vi "Split DMA by Direction.vi"(8 "error in":errorcluster, 11 "DMA configuration array":T1[](array[typedef])) -> (0 "error out":errorcluster, 2 "HostToTarget":T4[](array[typedef]) {"Data Type" format="%.0x"}, 3 "TargetToHost":T4[](array[typedef]) {"Data Type" format="%.0x"})   [LabVIEW 2018, in "FPGA Addon System Explorer.lvlib"]
uses:
  FPGA Addon System Explorer.lvlib
  Addon Shared/Types/DMA Information.ctl
  Addon Shared/Types/Data Type.ctl
  <vilib>/rvi/FIFO/Fifo_Types/Fifo_DMA_Config.ctl
  <vilib>/rvi/DataTransferAndStorage/Container/Common/niFpgaDataTypeControl.ctl
  <vilib>/rvi/ClientSDK/Core/ModuleGeneration/CommunicationInterfaceUtility/niFpgaDmaChannelImplementation.ctl
  Addon Shared/FPGA Addon Shared.lvlib
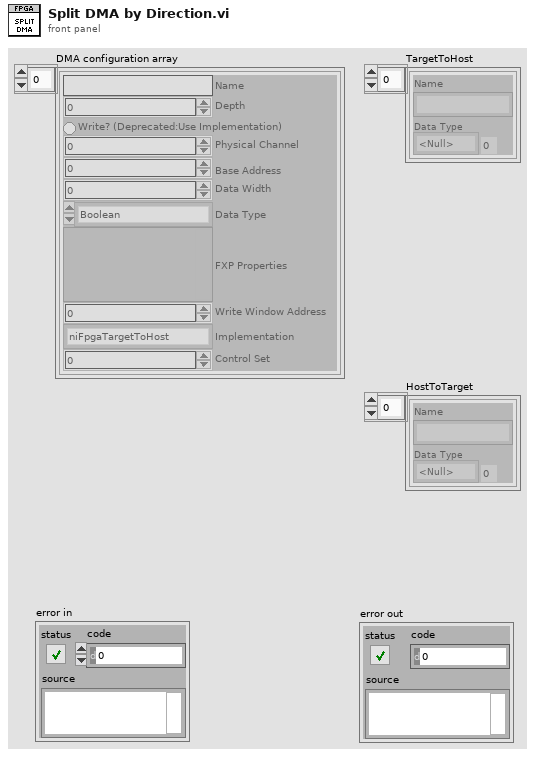
[diagram p1: front panel]
types:
  T1 = typedef "Fifo_DMA_Config.ctl" = cluster{"Name":string, "Depth":u32, "Write? (Deprecated:Use Implementation)":bool, "Physical Channel":u32, "Base Address":u32, "Data Width":u32, "Data Type":T2, "FXP Properties":variant, "Write Window Address":u32, "Implementation":T3, "Control Set":u32}
  T2 = typedef "niFpgaDataTypeControl.ctl" = enum32{"Boolean", "I8", "I16", "I32", "I64", "U8", "U16", "U32", "U64", "FXP", "CustomControl", "SGL"}
  T3 = typedef "niFpgaDmaChannelImplementation.ctl" = enum16{"niFpgaTargetToHost", "niFpgaHostToTarget", "niFpgaPeerToPeerWriter", "niFpgaPeerToPeerReader", "niCoreTargetToHost", "niCoreHostToTarget"}
  T4 = typedef "FPGA Addon Shared.lvlib/DMA Information.ctl" = cluster{"Name":string, "Data Type":T5}
  T5 = typedef "FPGA Addon Shared.lvlib/Data Type.ctl" = enum8{"<Null>", "I8", "I16", "I32", "I64", "U8", "U16", "U32", "U64", "SGL", "Boolean", "Analog PWM In Settings", "Analog PWM In", "Digital PWM In Settings", "Digital PWM In", "Digital PWM Out", "Sine Out", "FXP+/-24.5", "FXP+/-16.5", "FXP+/-32.8", "FXP+/-64.32", "FXP+/-16.7", "FXP+/-20.5", "FXP+/-27.5", "FXP+/-32.16", "FXP+16.3", "FXP+18.3", "Digital Static In", "Digital Static Out", "Digital Static In Settings", "Digital WSS Out", "Quad Encoder Settings", "Quad Encoder In", "Group"}
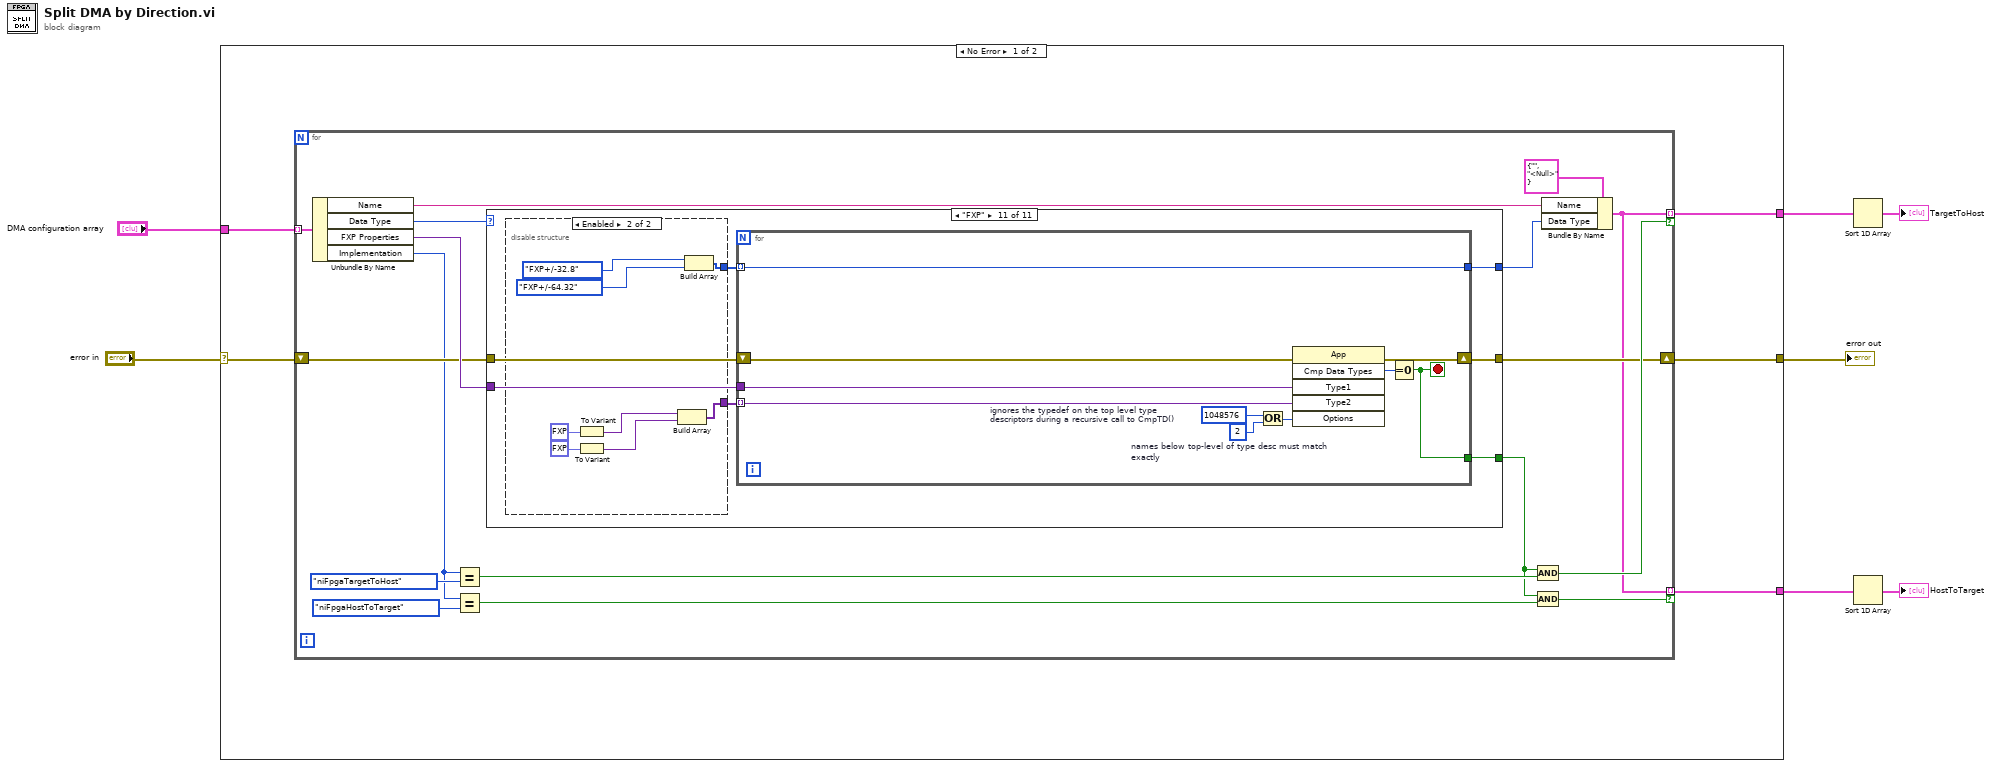
[diagram p0: block diagram]
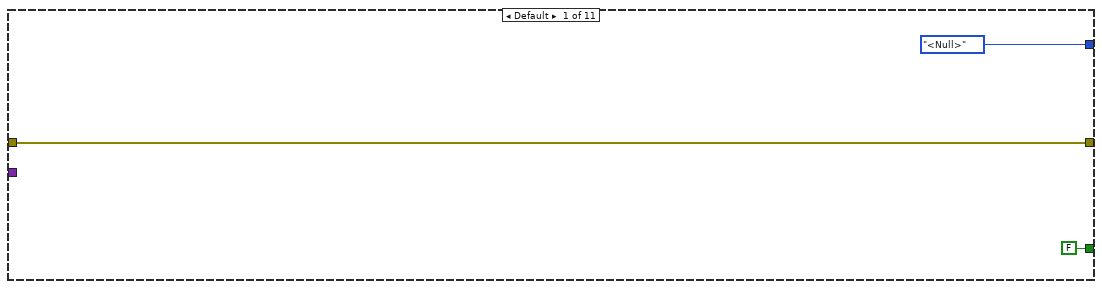
[diagram p2: hidden frame]
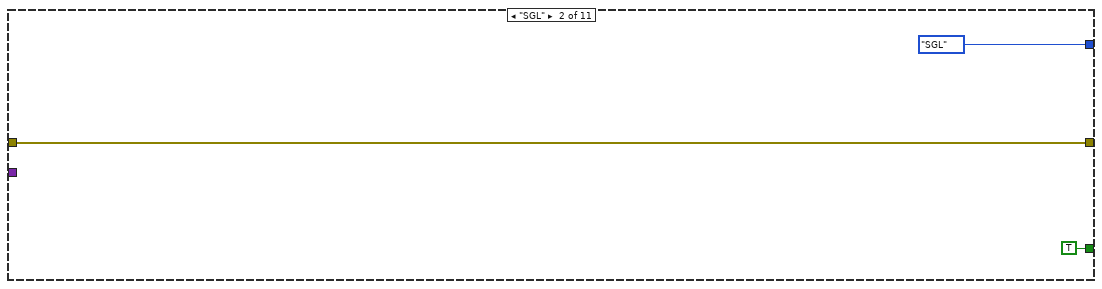
[diagram p3: hidden frame]
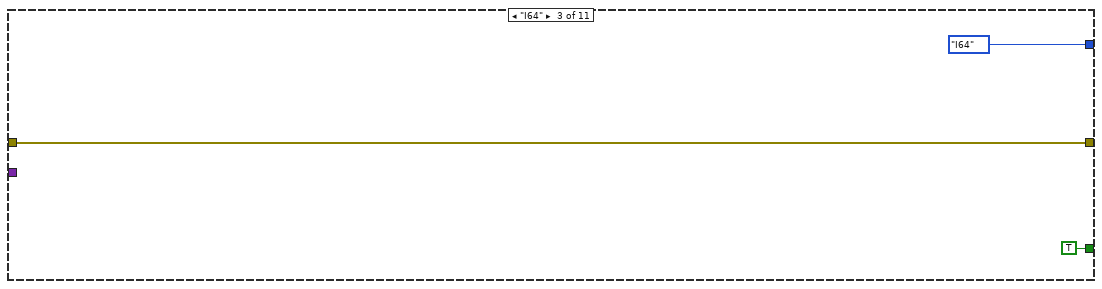
[diagram p4: hidden frame]
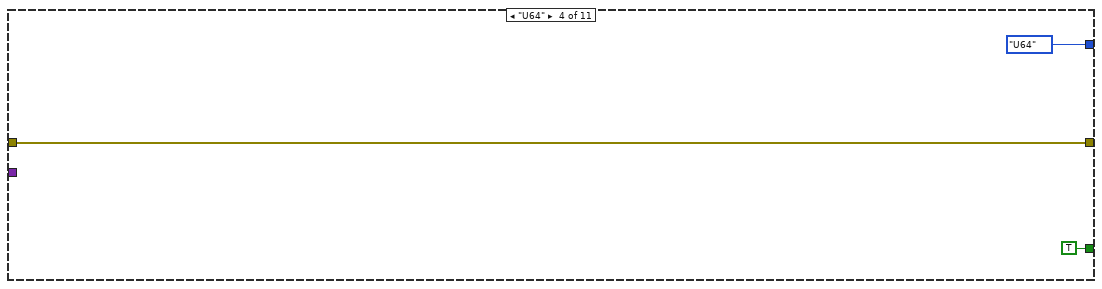
[diagram p5: hidden frame]
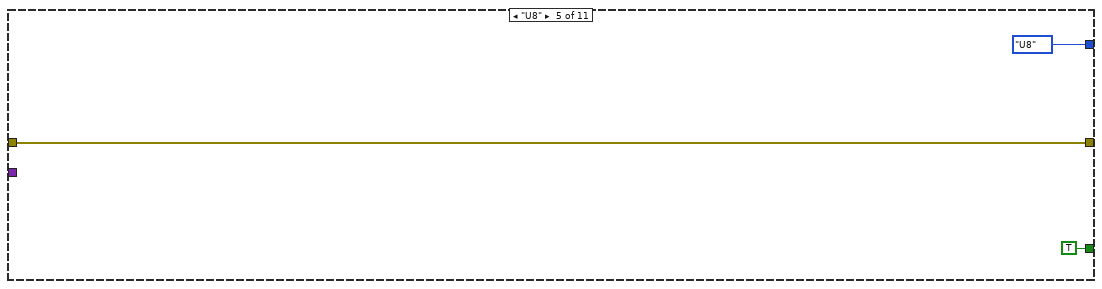
[diagram p6: hidden frame]
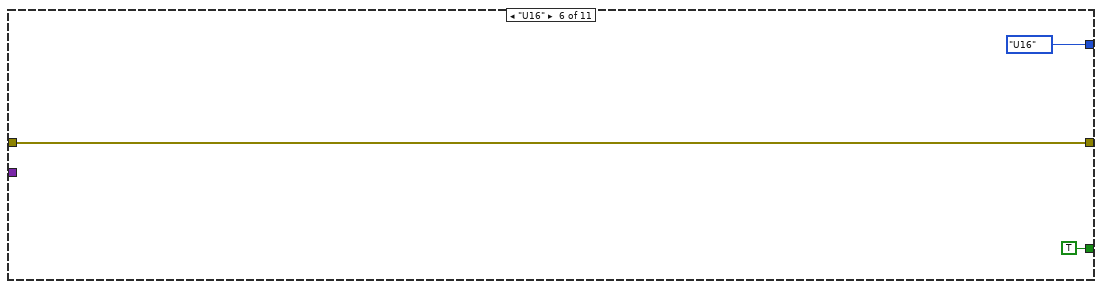
[diagram p7: hidden frame]
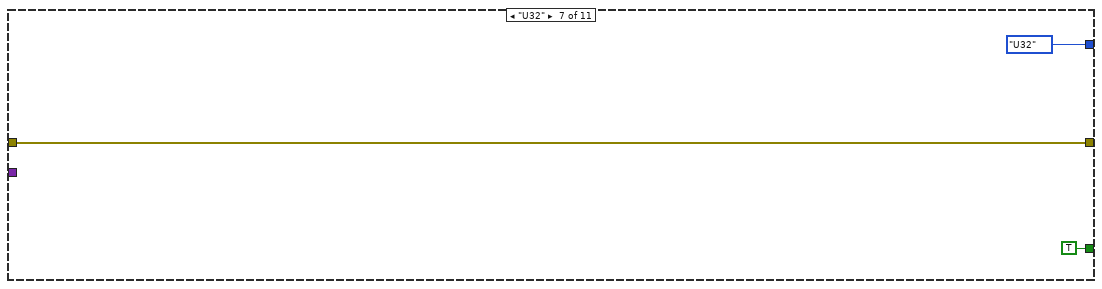
[diagram p8: hidden frame]
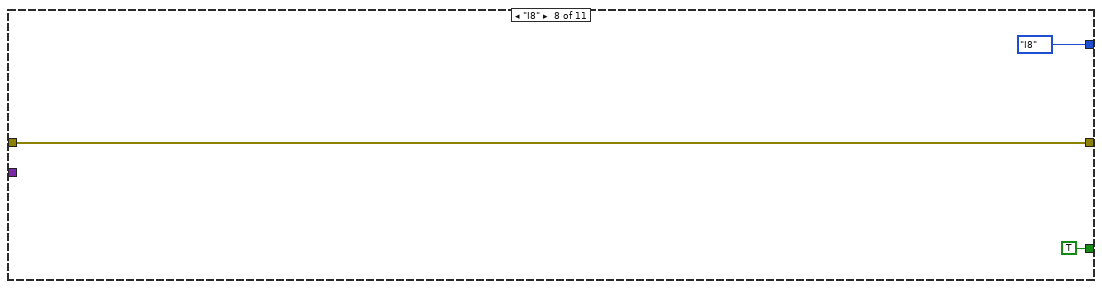
[diagram p9: hidden frame]
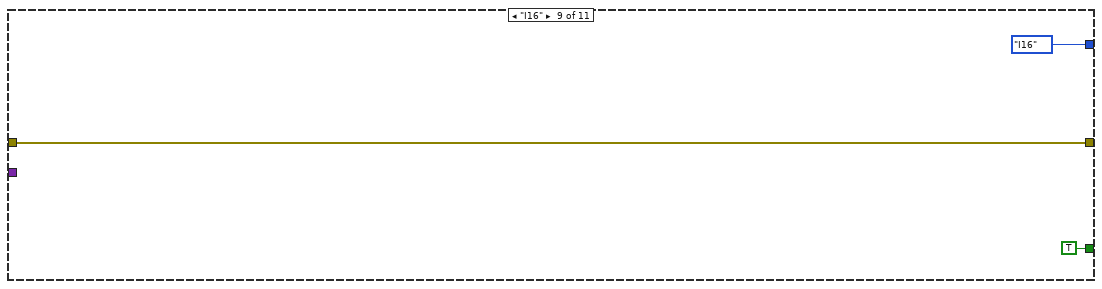
[diagram p10: hidden frame]
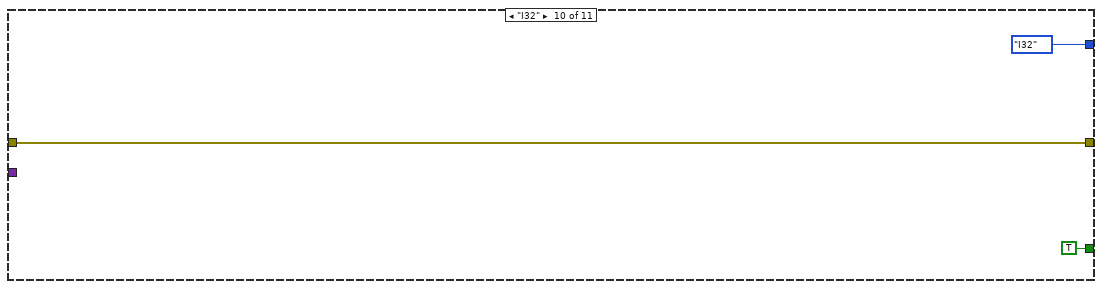
[diagram p11: hidden frame]
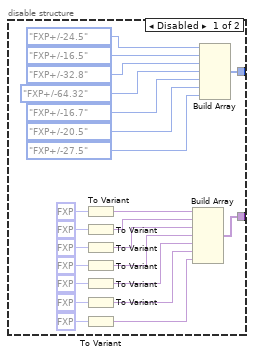
[diagram p12: hidden frame]
diagram:
  n1 = case shown="No Error" "error in" {
    selector: "error in" -> [w8 w108]
    tunnel: "DMA configuration array" -> [w12 _]
    tunnel: [w11 _] -> w5
    tunnel: [w10 _] -> w3
    tunnel: [w9 w108] -> w2
    frame No Error {
      n2 = for {
        tunnel: w12 -> [w15] mode=indexing
        tunnel: [w14] -> w10 mode=indexing if=w26
        tunnel: [w14] -> w11 mode=indexing if=w24
        shift-right: [w22] -> w9
        shift-left: w8 -> [w21]
        n3 = Unbundle By Name(w15) -> ("Name"=w19:string, "Data Type"=w18:T2, "FXP Properties"=w23:variant, "Implementation"=w13:T3)
        n4 = Equal?(x=w13, y=niFpgaDmaChannelImplementation."niFpgaTargetToHost") -> (x = y?=w27:bool)
        n5 = Equal?(x=w13, y=niFpgaDmaChannelImplementation."niFpgaHostToTarget") -> (x = y?=w25:bool)
        n6 = case shown="\"FXP\"" w18 {
          tunnel: w23 -> [_ _ _ _ _ _ _ _ _ _ w66]
          tunnel: [w32 w35 w38 w41 w44 w47 w50 w53 w56 w59 w65] -> w22
          tunnel: w21 -> [w32 w35 w38 w41 w44 w47 w50 w53 w56 w59 w64]
          tunnel: [Data_Type."<Null>" ("Data Type") Data_Type."SGL" ("Data Type") Data_Type."I64" ("Data Type") Data_Type."U64" ("Data Type") Data_Type."U8" ("Data Type") Data_Type."U16" ("Data Type") Data_Type."U32" ("Data Type") Data_Type."I8" ("Data Type") Data_Type."I16" ("Data Type") Data_Type."I32" ("Data Type") w61] -> w17
          tunnel: [FALSE TRUE TRUE TRUE TRUE TRUE TRUE TRUE TRUE TRUE w60] -> w16
          frame Default {
          }
          frame "SGL" {
          }
          frame "I64" {
          }
          frame "U64" {
          }
          frame "U8" {
          }
          frame "U16" {
          }
          frame "U32" {
          }
          frame "I8" {
          }
          frame "I16" {
          }
          frame "I32" {
          }
          frame "FXP" {
            n7 = disable-structure shown="Enabled" {
              disable-tunnel: [w75 w93] -> w63
              disable-tunnel: [w67 w90] -> w62
              frame Disabled {
                n8 = To Variant(anything=fxp<+/-,24,5> 0.0 ("Numeric 1 In")) -> (Variant=w76:variant)
                n9 = To Variant(anything=fxp<+/-,16,5> 0.0 ("Numeric 2 In")) -> (Variant=w77:variant)
                n10 = To Variant(anything=fxp<+/-,32,8> 0.0 ("Numeric 3 In")) -> (Variant=w78:variant)
                n11 = To Variant(anything=fxp<+/-,64,32> 0.0 ("Numeric 4 In")) -> (Variant=w79:variant)
                n12 = To Variant(anything=fxp<+/-,16,7> 0.0 ("Numeric 4 In")) -> (Variant=w85:variant)
                n13 = To Variant(anything=fxp<+/-,20,5> 0.0 ("Numeric 4 In")) -> (Variant=w87:variant)
                n14 = To Variant(anything=fxp<+/-,27,5> 0.0 ("Numeric 4 In")) -> (Variant=w89:variant)
                n15 = Build Array(w76, w77, w78, w79, w85, w87, w89) -> (w75:variant[])
                n16 = Build Array(Data_Type."FXP+/-24.5" ("Data Type"), Data_Type."FXP+/-16.5" ("Data Type"), Data_Type."FXP+/-32.8" ("Data Type"), Data_Type."FXP+/-64.32" ("Data Type"), Data_Type."FXP+/-16.7" ("Data Type"), Data_Type."FXP+/-20.5" ("Data Type"), Data_Type."FXP+/-27.5" ("Data Type")) -> (w67:T5[])
              }
              frame Enabled {
                n17 = To Variant(anything=fxp<+/-,32,8> 0.0 ("Numeric 3 In")) -> (Variant=w94:variant)
                n18 = To Variant(anything=fxp<+/-,64,32> 0.0 ("Numeric 4 In")) -> (Variant=w95:variant)
                n19 = Build Array(w94, w95) -> (w93:variant[])
                n20 = Build Array(Data_Type."FXP+/-32.8" ("Data Type"), Data_Type."FXP+/-64.32" ("Data Type")) -> (w90:T5[])
              }
            }
            n21 = for {
              tunnel: w66 -> [w103]
              tunnel: w63 -> [w102] mode=indexing
              shift-right: [w101] -> w65
              shift-left: w64 -> [w100]
              tunnel: w62 -> [w99] mode=indexing
              tunnel: [w99] -> w61
              tunnel: [w98] -> w60
              stop <- w98 stop-if-true
              w104 = 2  # names below top-level of type desc must match exactly
              w106 = 1048576  # ignores the typedef on the top level type descriptors during a recursive call to CmpTD()
              n22 = Or(x=w106, y=w104) -> (x .or. y?=w107:i32)
              n23 = invoke class="App" method="Cmp Data Types"(error in=w100, "Type1"=w103, "Type2"=w102, "Options"=w107) -> (error out=w101:errorcluster, "Compare Data Types"=w105:i32)  [unwired: 2 in, 4 out]
              n24 = Equal To 0?(x=w105) -> (x = 0?=w98:bool)
            }
          }
        }
        n25 = Compound Arithmetic op=AND(w16, w27) -> (w26:bool)
        n26 = Compound Arithmetic op=AND(w16, w25) -> (w24:bool)
        n27 = Bundle By Name(cluster=T4 {"Name"="", "Data Type"=enum."<Null>"} ("Cluster"), "Name"=w19, "Data Type"=w17) -> (w14:T4)
      }
    }
    frame Error {
    }
  }
  "error out" <- w2
  n28 = Sort 1D Array(array=w3) -> (sorted array=→"TargetToHost":T4[])
  n29 = Sort 1D Array(array=w5) -> (sorted array=→"HostToTarget":T4[])
